vi "Dictionary Test - 006.vi"(8 "error in (no error)":errorcluster) -> (0 "error out":errorcluster, 2 "pass":bool)   [LabVIEW 2009]
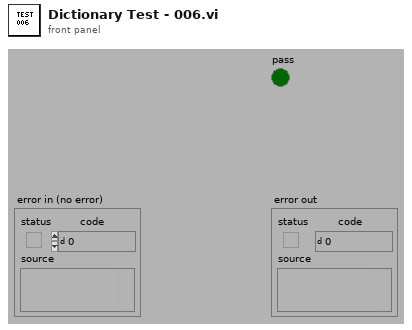
[diagram p1: front panel]
types:
  T1 = typedef "Dictionary Object RefNum.ctl" = refnum<k1>
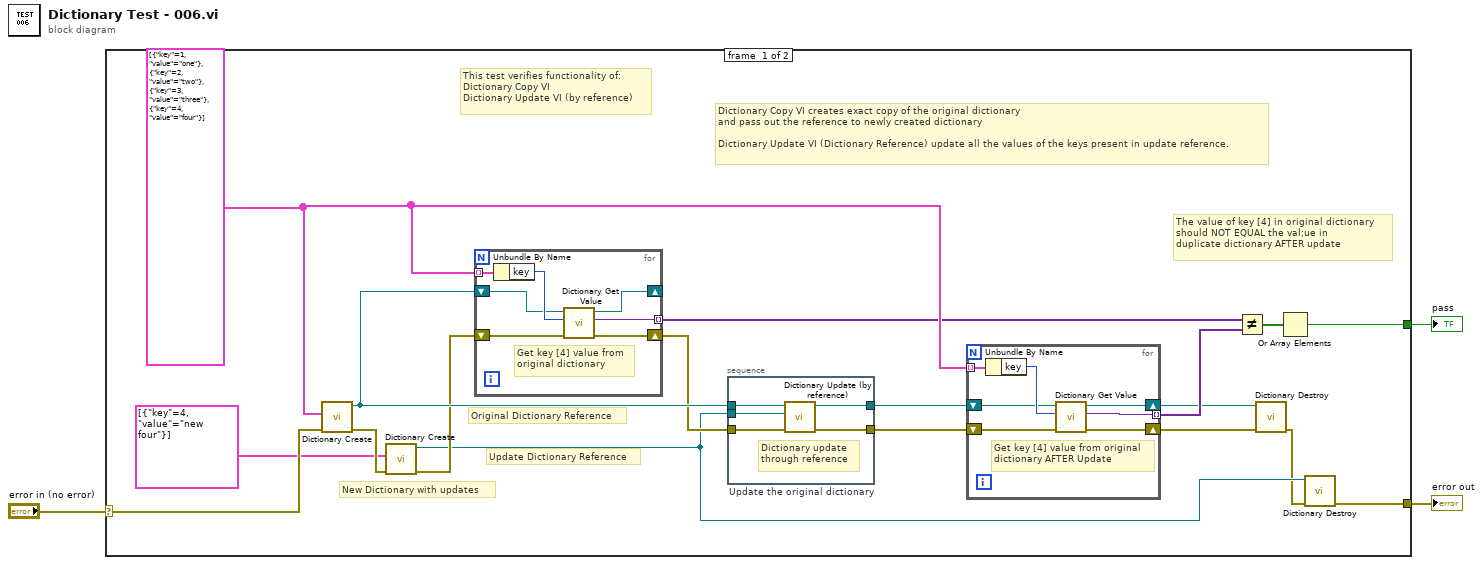
[diagram p0: block diagram]
diagram:
  n1 = case shown="No Error" "error in (no error)" {
    selector: "error in (no error)" -> [w15 w41]
    tunnel: [w5 w41] -> w2
    tunnel: [w7 _] -> w1
    frame #0 {
      w11 = cluster{"key":i32, "value":string}[] [{"key"=1, "value"="one"}, {"key"=2, "value"="two"}, {"key"=3, "value"="three"}, {"key"=4, "value"="four"}] ("dictionary with updates")
      # "New Dictionary with updates"
      # "Original Dictionary Reference"
      # "Update Dictionary Reference"
      # "The value of key [4] in original dictionary\nshould NOT EQUAL the val;ue in \nduplicate dictionary AFTER update"
      # "Dictionary Copy VI creates exact copy of the original dictionary \nand pass out the reference to newly created dictionary\n\nDictionary Update VI (Dictionary Reference) update all the values of the keys present in update reference."
      # "This test verifies functionality of:\nDictionary Copy VI\nDictionary Update VI (by reference)"
      n2 = call "Dictionary Create.vi"("error in (no error)"=w15, "initial dictionary (empty)"=w11) -> ("error out"=w14:errorcluster, "dictionary out"=w21:T1)  [unwired: 8 in]
      n3 = call "Dictionary Create.vi"("error in (no error)"=w14, "initial dictionary (empty)"=cluster{"key":i32, "value":string}[] [{"key"=4, "value"="new four"}]) -> ("error out"=w13:errorcluster, "dictionary out"=w6:T1)  [unwired: 8 in]
      n4 = for {
        tunnel: [w35] -> w10 mode=indexing
        tunnel: w11 -> [w34] mode=indexing
        shift-right: [w32] -> _
        shift-left: w21 -> [w31]
        shift-right: [w30] -> w12
        shift-left: w13 -> [w29]
        # "Get key [4] value from\noriginal dictionary"
        n5 = Unbundle By Name(w34) -> ("key"=w33:i32)
        n6 = call "Dictionary Get Value.vi"("error in"=w29, "key"=w33, "dictionary"=w31) -> ("error out"=w30:errorcluster, "value"=w35:variant, "dictionary out"=w32:T1)  [unwired: 5 in, 1 out]
      }
      n7 = stacked-sequence "Update the original dictionary" {
        tunnel: [w40] -> w20
        tunnel: [w39] -> w19
        tunnel: w12 -> [w38]
        tunnel: w21 -> [w37]
        tunnel: w6 -> [w36]
        frame #0 {
          # "Dictionary update \nthrough reference"
          n8 = call "Dictionary Update (by reference).vi"("error in (no error)"=w38, "dictionary with updates"=w36, "dictionary"=w37) -> ("error out"=w39:errorcluster, "dictionary out"=w40:T1)  [unwired: 6 in, 1 out]
        }
      }
      n9 = for {
        tunnel: [w28] -> w18 mode=indexing
        tunnel: w11 -> [w27] mode=indexing
        shift-right: [w25] -> w17
        shift-left: w20 -> [w24]
        shift-right: [w23] -> w16
        shift-left: w19 -> [w22]
        # "Get key [4] value from original\ndictionary AFTER Update"
        n10 = Unbundle By Name(w27) -> ("key"=w26:i32)
        n11 = call "Dictionary Get Value.vi"("error in"=w22, "key"=w26, "dictionary"=w24) -> ("error out"=w23:errorcluster, "value"=w28:variant, "dictionary out"=w25:T1)  [unwired: 5 in, 1 out]
      }
      n12 = Not Equal?(x=w10, y=w18) -> (x != y?=w9:bool[])
      n13 = call "Dictionary Destroy.vi"("error in (no error)"=w16, "dictionary"=w17) -> ("error out"=w4:errorcluster)  [unwired: 9 in]
      n14 = Or Array Elements(Boolean array=w9) -> (logical OR=w7:bool)
      n15 = call "Dictionary Destroy.vi"("error in (no error)"=w4, "dictionary"=w6) -> ("error out"=w5:errorcluster)  [unwired: 9 in]
    }
    frame #1 {
    }
  }
  "pass" <- w1
  "error out" <- w2
